vi "get move settings calb.vi"(8 "error in (no error)":errorcluster, 9 "calibration":cluster{"A":dbl, "MicrostepMode":u32}, 10 "move_settings_calb":T1, 11 "id":i32) -> (0 "error out":errorcluster, 2 "move_settings_calb out":T1, 3 "function return":i32)   [LabVIEW 2012, in "libximc.lvlib"]
doc: "result_t XIMC_API get_move_settings_calb (device_t id, move_settings_calb_t* move_settings_calb, const calibration_t* calibration);"
uses:
  libximc.lvlib
  libximc.dll
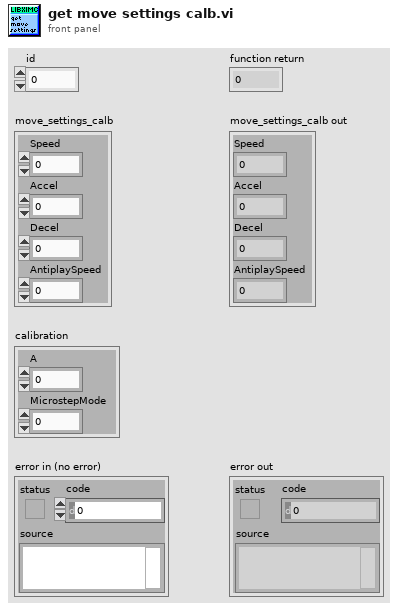
[diagram p1: front panel]
types:
  T1 = cluster{"Speed":sgl, "Accel":sgl, "Decel":sgl, "AntiplaySpeed":sgl}
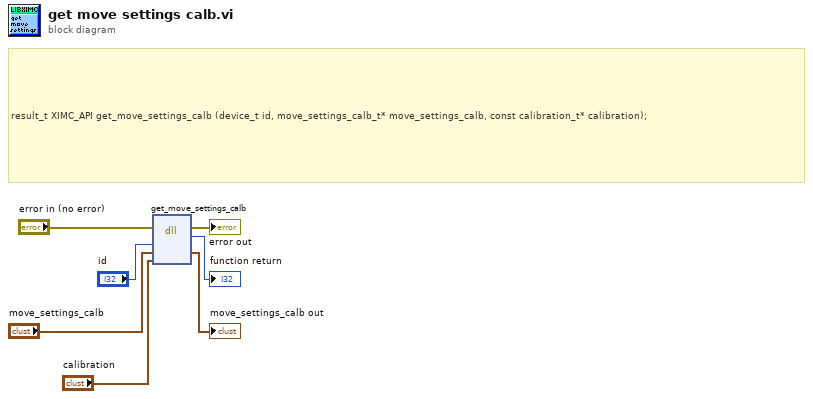
[diagram p0: block diagram]
diagram:
  # "result_t XIMC_API get_move_settings_calb (device_t id, move_settings_calb_t* move_settings_calb, const calibration_t* calibration);"
  n1 = dll-call lib="C:/Users/Vasily/Att_examples/LabVIEW_example/libximc.*" fn="get_move_settings_calb"(error in="error in (no error)", "id"="id", "move_settings_calb"="move_settings_calb", "calibration"="calibration") -> (error out=→"error out":errorcluster, →"function return":i32, "move_settings_calb"=→"move_settings_calb out":T1)  [unwired: 4 in, 1 out]
